vi "Util_Progress Show Progress Popup with Status.vi"(7 "Deployment Notifiers":T1, 8 "error in (no error)":errorcluster, 9 "Title":string, 10 "Message":string) -> (0 "error out":errorcluster)   [LabVIEW 2016]
uses:
  App Images/TypeDefs/rad_Deployment Notifiers.ctl
  App Images/TypeDefs/rad_Deployment Status Data Type.ctl
  App Images/TypeDefs/rad_Deployment Progress Data Type.ctl
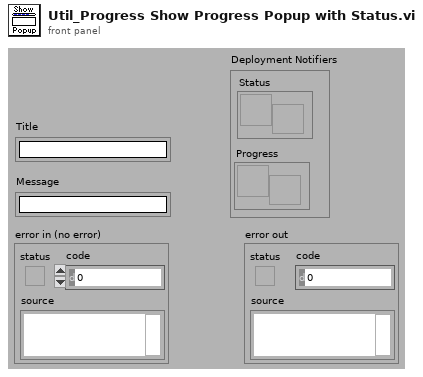
[diagram p1: front panel]
types:
  T1 = typedef "rad_Deployment Notifiers.ctl" = cluster{"Status":refnum<notifier>, "Progress":refnum<notifier>}
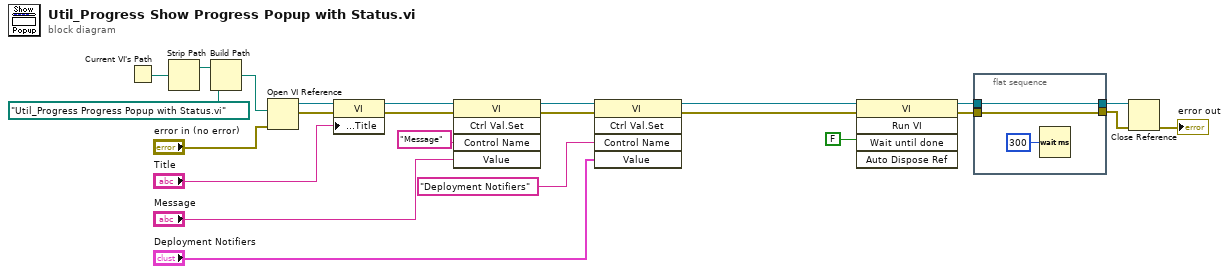
[diagram p0: block diagram]
diagram:
  n1 = Current VI's Path() -> (path=w14:path)
  n2 = Strip Path(path=w14) -> (stripped path=w13:path)  [unwired: 1 out]
  n3 = Build Path(base path=w13, name or relative path=path "Util_Progress Progress Popup with Status.vi" ("vi path")) -> (appended path=w11:path)
  n4 = Open VI Reference(vi path=w11, error in (no error)="error in (no error)") -> (vi reference=w23:refnum<vi>, error out=w24:errorcluster)  [unwired: 4 out]
  n5 = property class="VI"(reference=w23, error in=w24, "Front Panel.Title"="Title") -> (reference out=w18:refnum<vi>, error out=w19:errorcluster)
  n6 = invoke class="VI" method="Ctrl Val.Set"(reference=w18, error in=w19, "Control Name"="Message", "Value"="Message") -> (reference out=w6:refnum<vi>, error out=w5:errorcluster)  [unwired: 1 in, 3 out]
  n7 = invoke class="VI" method="Ctrl Val.Set"(reference=w6, error in=w5, "Control Name"="Deployment Notifiers", "Value"="Deployment Notifiers") -> (reference out=w2:refnum<vi>, error out=w1:errorcluster)  [unwired: 1 in, 3 out]
  n8 = invoke class="VI" method="Run VI"(reference=w2, error in=w1, "Wait until done"=FALSE ("Wait Until Done")) -> (reference out=w7:refnum<vi>, error out=w10:errorcluster)  [unwired: 2 in, 3 out]
  n9 = flat-sequence {
    tunnel: [w27] -> w9
    tunnel: w10 -> [w27]
    tunnel: w7 -> [w26]
    tunnel: [w26] -> w8
    frame #0 {
      n10 = Wait (ms)(milliseconds to wait=u32 300) -> ()  [unwired: 1 out]
    }
  }
  n11 = Close Reference(reference=w8, error in (no error)=w9) -> (error out=→"error out":errorcluster)
